vi "sub_wfm-buffer.vi"(7 "cmd":T1, 8 "data":dbl[](array[numeric]), 9 "inx":i32, 10 "history size":i32=60, 11 "dim":i32=730) -> (3 "Array":dbl[][](array[numeric]))   [LabVIEW 2021]
uses:
  ctrl/init-r-update.ctl
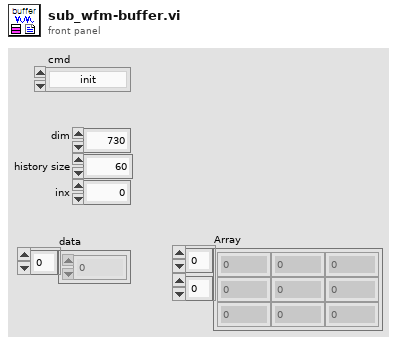
[diagram p1: front panel]
types:
  T1 = typedef "init-r-update.ctl" = enum16{"init", "read", "update"}
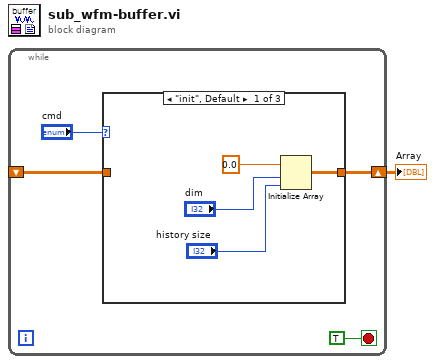
[diagram p0: block diagram]
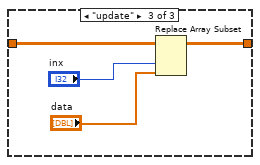
[diagram p3: hidden frame]
diagram:
  n1 = while {
    shift-right: [w3] -> w1
    shift-left: _ -> [w2]
    stop <- TRUE stop-if-true
    n2 = case shown="\"init\", Default" "cmd" {
      tunnel: [w6 w10 w13] -> w3
      tunnel: w2 -> [_ w10 w14]
      frame "init", Default {
        n3 = Initialize Array(0.0 ("element"), "dim", "history size") -> (w6:dbl[][])
      }
      frame "read" {
      }
      frame "update" {
        n4 = Replace Array Subset(array=w14, new element="data", index (col)="inx") -> (w13:dbl[][])  [unwired: 1 in]
      }
    }
  }
  "Array" <- w1
